vi "Digital_Input_4Channels.vi"(1 "IO":T1={"DI 0"="Mod1/DIO2", "DI 1"="Mod1/DIO2", "DI 2"="Mod1/DIO2", "DI 3"="Mod1/DIO2"}) -> (0 "States":bool[](array[boolean]))   [LabVIEW 2015]
uses:
  <vilib>/rvi/eio/common/nirviEmuTemplateMethod_errors.vi
  <vilib>/eio/EIONode/EIONode.xnode
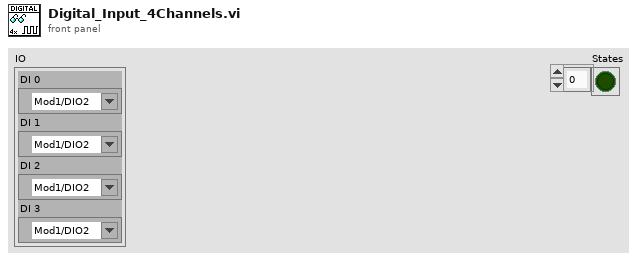
[diagram p1: front panel]
types:
  T1 = cluster{"DI 0":refnum<k21>, "DI 1":refnum<k21>, "DI 2":refnum<k21>, "DI 3":refnum<k21>}
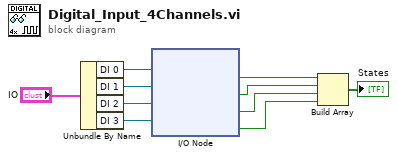
[diagram p0: block diagram]
diagram:
  n1 = Unbundle By Name("IO") -> ("DI 0"=w9:refnum<k21>, "DI 1"=w8:refnum<k21>, "DI 2"=w7:refnum<k21>, "DI 3"=w6:refnum<k21>)
  n2 = xnode "I/O Node"("FPGA I/O In"=w9, "FPGA I/O In"=w8, "FPGA I/O In"=w7, "FPGA I/O In"=w6) -> ("I/O Item"=w5:bool, "I/O Item"=w4:bool, "I/O Item"=w3:bool, "I/O Item"=w2:bool)  [unwired: 4 out]
  n3 = Build Array(w5, w4, w3, w2) -> (→"States":bool[])
